vi "NET_System_States.vi"(8 "Read(F) Write(T)":bool, 9 "Lift State In":T1, 10 "Claw Rotation State In":T2, 11 "Arm State In":T3) -> (1 "Lift State Out":T1, 2 "Claw Rotation State Out":T2, 3 "Arm State Out":T3)   [LabVIEW 2017]
uses:
  RoboRio Code/Systems/Arm/ENUM_SM_State.ctl
  RoboRio Code/Systems/Claw Rotation/ENUM_SM_State.ctl
  RoboRio Code/Systems/Lift/ENUM_SM_State.ctl
  <vilib>/Rock Robotics/Network Tables/NT Read Numeric Array.vi
  <vilib>/Rock Robotics/Network Tables/NT Write Numeric Array.vi
  RoboRio Code/Systems/Arm/Arm.lvlib
  RoboRio Code/Systems/Claw Rotation/Claw_Rotation.lvlib
  RoboRio Code/Systems/Lift/Lift.lvlib
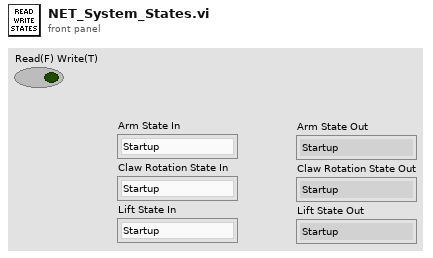
[diagram p1: front panel]
types:
  T1 = typedef "Lift.lvlib/ENUM_SM_State.ctl" = enum16{"Startup", "Idle", "F_Manual", "Manual", "Position - Moving", "Position - Holding", "Shutdown"}
  T2 = typedef "Claw_Rotation.lvlib/ENUM_SM_State.ctl" = enum16{"Startup", "Idle", "F_Manual", "Manual", "Position - Moving", "Position - Holding", "Shutdown"}
  T3 = typedef "Arm.lvlib/ENUM_SM_State.ctl" = enum16{"Startup", "Idle", "F_Manual", "Manual", "Position - Moving", "Position - Holding", "Shutdown"}
  T4 = cluster{"Arm State In":T3, "Claw Rotation State In":T2, "Lift State In":T1}
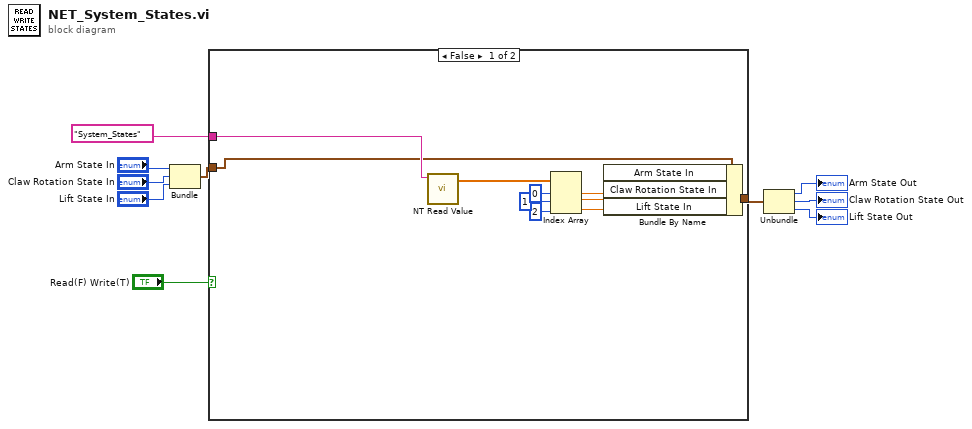
[diagram p0: block diagram]
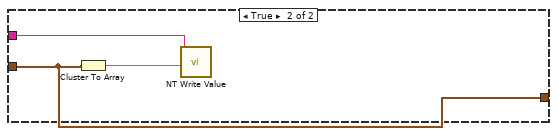
[diagram p2: hidden frame]
diagram:
  n1 = Bundle("Arm State In"="Arm State In", "Claw Rotation State In"="Claw Rotation State In", "Lift State In"="Lift State In") -> (w8:T4)  [unwired: 1 in]
  n2 = case shown="False" "Read(F) Write(T)" {
    tunnel: "System_States" ("Name") -> [w20 w23]
    tunnel: w8 -> [w15 w21]
    tunnel: [w14 w21] -> w4
    frame False {
      n3 = call-poly <vilib>:"NT Read Value.vi"("Name"=w20) -> ("Numeric Array"=w19:dbl[])  [unwired: 9 in, 1 out]
      n4 = Index Array(array=w19, index #1=0 ("index"), index #2=1 ("index"), index #3=2 ("index")) -> (element #1=w13:dbl, element #2=w12:dbl, element #3=w11:dbl)
      n5 = Bundle By Name(cluster=w15, "Arm State In"=w13, "Claw Rotation State In"=w12, "Lift State In"=w11) -> (w14:T4)
    }
    frame True {
      n6 = Cluster To Array(cluster=w21) -> (array=w22:T1[])
      n7 = call-poly <vilib>:"NT Write Value.vi"("Numeric Array"=w22, "Name"=w23) -> ()  [unwired: 9 in, 1 out]
    }
  }
  n8 = Unbundle(w4) -> ("Arm State In"=→"Arm State Out":T3, "Claw Rotation State In"=→"Claw Rotation State Out":T2, "Lift State In"=→"Lift State Out":T1)
